vi "Input_Auth_Code.vi"() -> (0 "Code Out":string)   [LabVIEW 2016]
panel:
  in  "?":bool
  in  "Authorization Code":string
  # "From the browser window, please get the code out of the URL that you are redirected to.\nIt will be in the form [url]&code={code}\nThis code should be a string of letters and numbers."
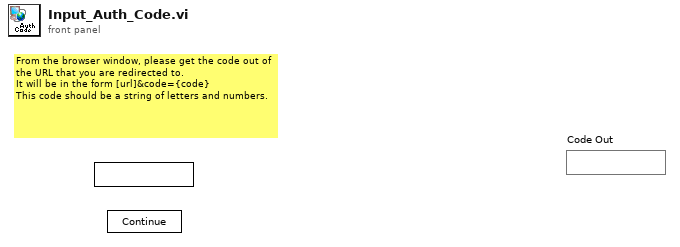
[diagram p1: front panel]
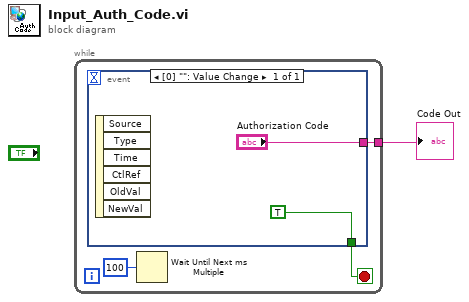
[diagram p0: block diagram]
diagram:
  n1 = while {
    tunnel: [w2] -> w1
    stop <- w4 stop-if-true
    n2 = event shown="[0] \"\": Value Change" {
      selector: _ -> [_]
      dyn-events: _ -> [_]
      timeout: _ -> [_]
      tunnel: [TRUE] -> w4
      tunnel: ["Authorization Code"] -> w2
      event Value Change {
        n3 = event-data() -> ()  [unwired: 1 in, 6 out]
      }
    }
    n4 = Wait Until Next ms Multiple(millisecond multiple=u32 100) -> ()  [unwired: 1 out]
  }
  "Code Out" <- w1
